vi "17_1.vi"() -> ()   [LabVIEW 2018]
panel:
  out "sum":i16
  out "Array 2":bool[][][](array[boolean])
  in  "Input":string
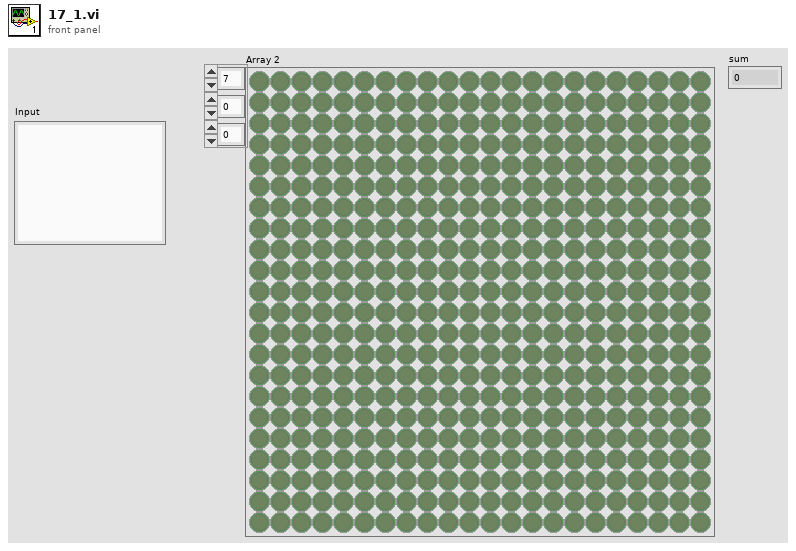
[diagram p1: front panel]
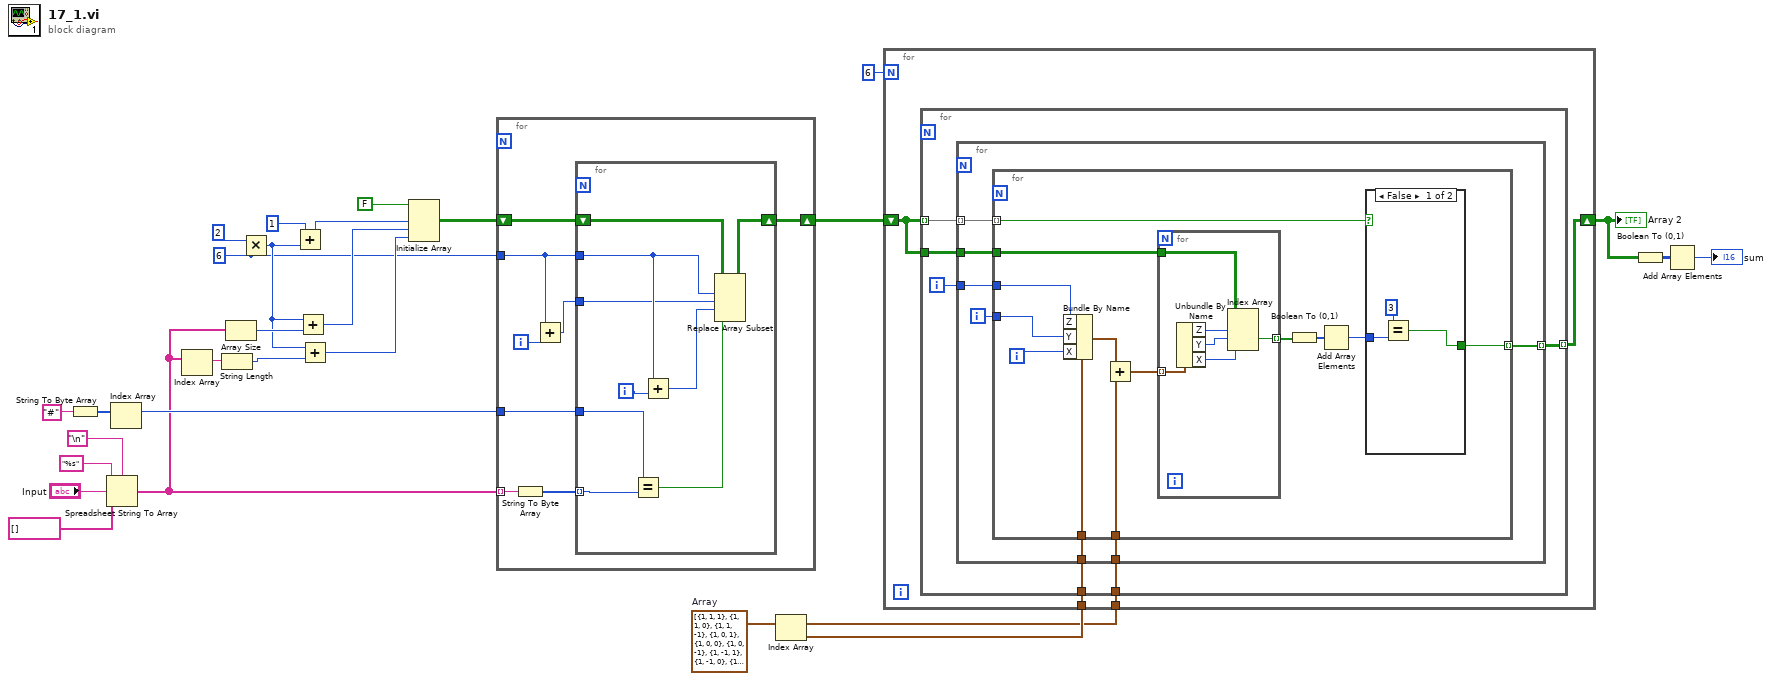
[diagram p0: block diagram]
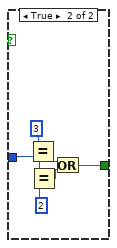
[diagram p2: hidden frame]
diagram:
  w5 = cluster{"Z":i32, "Y":i32, "X":i32}[] [{"Z"=1, "Y"=1, "X"=1}, {"Z"=1, "Y"=1, "X"=0}, {"Z"=1, "Y"=1, "X"=-1}, {"Z"=1, "Y"=0, "X"=1}, {"Z"=1, "Y"=0, "X"=0}, {"Z"=1, "Y"=0, "X"=-1}, {"Z"=1, "Y"=-1, "X"=1}, {"Z"=1, "Y"=-1, "X"=0}, {"Z"=1, "Y"=-1, "X"=-1}, {"Z"=0, "Y"=1, "X"=1}, {"Z"=0, "Y"=1, "X"=0}, {"Z"=0, "Y"=1, "X"=-1}, {"Z"=0, "Y"=0, "X"=1}, {"Z"=0, "Y"=0, "X"=-1}, {"Z"=0, "Y"=-1, "X"=1}, {"Z"=0, "Y"=-1, "X"=0}, {"Z"=0, "Y"=-1, "X"=-1}, {"Z"=-1, "Y"=1, "X"=1}, {"Z"=-1, "Y"=1, "X"=0}, {"Z"=-1, "Y"=1, "X"=-1}, {"Z"=-1, "Y"=0, "X"=1}, {"Z"=-1, "Y"=0, "X"=0}, {"Z"=-1, "Y"=0, "X"=-1}, {"Z"=-1, "Y"=-1, "X"=1}, {"Z"=-1, "Y"=-1, "X"=0}, {"Z"=-1, "Y"=-1, "X"=-1}]  # Array
  w8 = 6
  n1 = String To Byte Array(string="#") -> (unsigned byte array=w22:u8[])
  n2 = Spreadsheet String To Array(delimiter (Tab)="\n", format string="%s", spreadsheet string="Input", array type (2D Dbl)=string[] []) -> (array=w14:string[])
  n3 = Index Array(array=w22) -> (element=w21:u8)  [unwired: 1 in]
  n4 = Index Array(array=w14) -> (element=w13:string)  [unwired: 1 in]
  n5 = String Length(string=w13) -> (length=w12:i32)
  n6 = Array Size(array=w14) -> (size(s)=w19:i32)
  n7 = Multiply(x=2, y=w8) -> (x*y=w11:i32)
  n8 = Add(x=1, y=w11) -> (x+y=w17:i32)
  n9 = Add(x=w11, y=w19) -> (x+y=w15:i32)
  n10 = Add(x=w11, y=w12) -> (x+y=w10:i32)
  n11 = Initialize Array(FALSE, w17, w15, w10) -> (w9:bool[][][])
  n12 = for {
    tunnel: w14 -> [w35] mode=indexing
    tunnel: w21 -> [w33]
    shift-right: [w31] -> w7
    shift-left: w9 -> [w32]
    tunnel: w8 -> [w29]
    i -> [w30]
    n13 = String To Byte Array(string=w35) -> (unsigned byte array=w34:u8[])
    n14 = Add(x=w29, y=w30) -> (x+y=w28:i32)
    n15 = for {
      tunnel: w34 -> [w44] mode=indexing
      tunnel: w33 -> [w43]
      shift-right: [w41] -> w31
      shift-left: w32 -> [w42]
      tunnel: w29 -> [w38]
      tunnel: w28 -> [w36]
      i -> [w39]
      n16 = Equal?(x=w43, y=w44) -> (x = y?=w40:bool)
      n17 = Add(x=w38, y=w39) -> (x+y=w37:i32)
      n18 = Replace Array Subset(array=w42, new element=w40, index (dim 0)=w38, index (dim 1)=w36, index (dim 2)=w37) -> (w41:bool[][][])
    }
  }
  n19 = Index Array(array=w5) -> (element=w6:cluster{"Z":i32, "Y":i32, "X":i32})  [unwired: 1 in]
  n20 = for {
    N: 6 -> [_]
    tunnel: w6 -> [w48]
    tunnel: w5 -> [w47]
    shift-right: [w46] -> w2
    shift-left: w7 -> [w45]
    n21 = for {
      tunnel: w45 -> [w54] mode=indexing
      tunnel: w45 -> [w53]
      tunnel: w48 -> [w52]
      tunnel: w47 -> [w50]
      tunnel: [w49] -> w46 mode=indexing
      i -> [w51]
      n22 = for {
        tunnel: w54 -> [w61] mode=indexing
        tunnel: w53 -> [w60]
        tunnel: w52 -> [w59]
        tunnel: w51 -> [w57]
        tunnel: w50 -> [w56]
        tunnel: [w55] -> w49 mode=indexing
        i -> [w58]
        n23 = for {
          tunnel: w61 -> [w66] mode=indexing
          tunnel: w60 -> [w67]
          tunnel: w59 -> [w74]
          tunnel: w58 -> [w72]
          tunnel: w57 -> [w71]
          tunnel: w56 -> [w69]
          tunnel: [w62] -> w55 mode=indexing
          i -> [w73]
          n24 = Bundle By Name(cluster=w74, "Z"=w71, "Y"=w72, "X"=w73) -> (w70:cluster{"Z":i32, "Y":i32, "X":i32})
          n25 = Add(x=w70, y=w69) -> (x+y=w68:cluster{"Z":i32, "Y":i32, "X":i32}[])
          n26 = for {
            tunnel: w68 -> [w88] mode=indexing
            tunnel: w67 -> [w89]
            tunnel: [w84] -> w65 mode=indexing
            n27 = Unbundle By Name(w88) -> ("Z"=w87:i32, "Y"=w86:i32, "X"=w85:i32)
            n28 = Index Array(array=w89, index (dim 0)=w87, index (dim 1)=w86, index (dim 2)=w85) -> (element=w84:bool)
          }
          n29 = Boolean To (0,1)(Boolean=w65) -> (0, 1=w64:i16[])
          n30 = Add Array Elements(numeric array=w64) -> (sum=w63:i16)
          n31 = case shown="False" w66 {
            tunnel: w63 -> [w76 w83]
            tunnel: [w75 w78] -> w62
            frame False {
              n32 = Equal?(x=i16 3, y=w76) -> (x = y?=w75:bool)
            }
            frame True {
              n33 = Equal?(x=i16 3, y=w83) -> (x = y?=w80:bool)
              n34 = Equal?(x=w83, y=i16 2) -> (x = y?=w79:bool)
              n35 = Or(x=w80, y=w79) -> (x .or. y?=w78:bool)
            }
          }
        }
      }
    }
  }
  "Array 2" <- w2
  n36 = Boolean To (0,1)(Boolean=w2) -> (0, 1=w3:i16[][][])
  n37 = Add Array Elements(numeric array=w3) -> (sum=→"sum":i16)
